vi "FindSimETH_CF.vi"(6 "COM":string, 8 "error in (no error)":errorcluster) -> (0 "error out":errorcluster, 1 "Pass":bool, 2 "CmdOut":string)   [LabVIEW 2013]
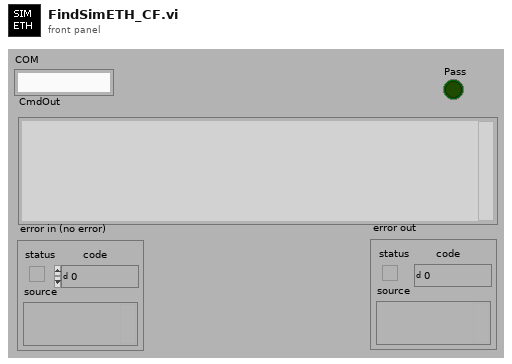
[diagram p1: front panel]
types:
  T1 = enum32{"invalid app kind", "Development System", "Run Time System", "Student Edition", "Embedded LabVIEW", "Evaluation", "Custom"}
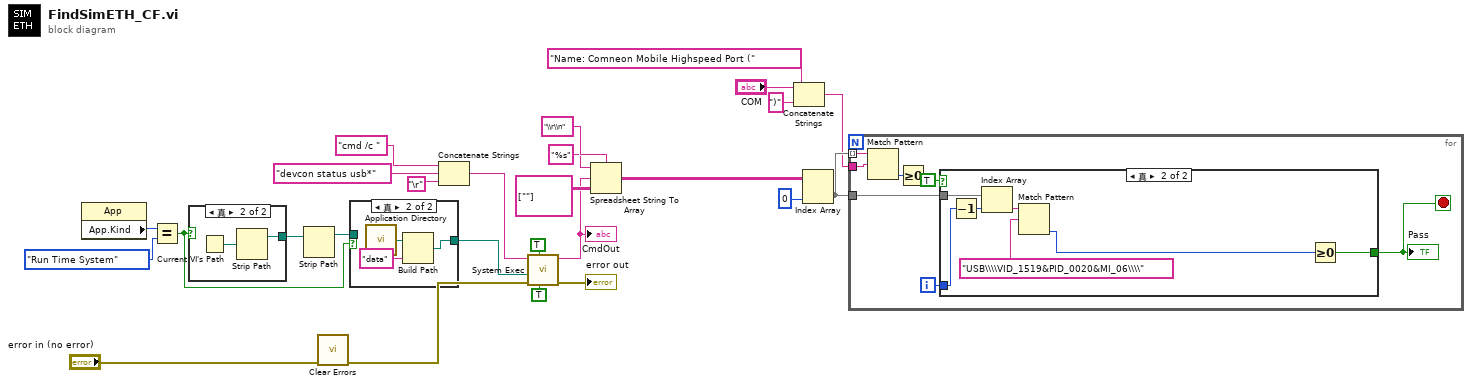
[diagram p0: block diagram]
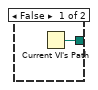
[diagram p3: hidden frame]
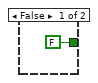
[diagram p4: hidden frame]
diagram:
  n1 = property class="App"() -> ("App.Kind"=w13:T1)  [unwired: 2 in, 2 out]
  n2 = Equal?(x=w13, y=T1."Run Time System") -> (x = y?=w4:bool)
  n3 = case shown="真" w4 {
    tunnel: [w27 w29] -> w12
    frame False {
      n4 = Current VI's Path() -> (path=w27:path)
    }
    frame True {
      n5 = Current VI's Path() -> (path=w28:path)
      n6 = Strip Path(path=w28) -> (stripped path=w29:path)  [unwired: 1 out]
    }
  }
  n7 = Strip Path(path=w12) -> (stripped path=w5:path)  [unwired: 1 out]
  n8 = call <vilib>:"Clear Errors.vi"("error in (no error)"="error in (no error)") -> ("error out"=w2:errorcluster)  [unwired: 6 in]
  n9 = case shown="真" w4 {
    tunnel: w5 -> [w30 _]
    tunnel: [w30 w31] -> w1
    frame False {
    }
    frame True {
      n10 = call <vilib>:"Application Directory.vi"() -> ("Application Directory"=w33:path)
      n11 = Build Path(base path=w33, name or relative path="data" ("名称或相对路径")) -> (appended path=w31:path)
    }
  }
  n12 = Concatenate Strings("cmd /c " ("command line"), "devcon status usb*" ("command"), "\r") -> (w24:string)
  n13 = call <vilib>:"System Exec.vi"("run minimized? (F)"=TRUE, "wait until completion? (T)"=TRUE, "error in (no error)"=w2, "working directory"=w1, "command line"=w24) -> ("error out"=→"error out":errorcluster, "standard output"=w15:string)  [unwired: 1 in, 4 out]
  "CmdOut" <- w15
  n14 = Spreadsheet String To Array(delimiter (Tab)="\\r\\n" ("格式字符串"), format string="%s" ("格式字符串"), spreadsheet string=w15, array type (2D Dbl)=string[][] [[""]]) -> (array=w17:string[][])
  n15 = Concatenate Strings("Name: Comneon Mobile Highspeed Port (" ("command line"), "COM", ")" ("字符串")) -> (w7:string)
  n16 = Index Array(array=w17, index (col)=0 ("索引 (行)")) -> (element=w10:string[])  [unwired: 1 in]
  n17 = for {
    tunnel: w10 -> [w40] mode=indexing
    tunnel: w7 -> [w39]
    tunnel: w10 -> [w37]
    i -> [w38]
    stop <- w35 stop-if-true
    n18 = Match Pattern(string=w40, regular expression=w39) -> (offset past match=w36:i32)  [unwired: 4 out]
    n19 = Greater Or Equal To 0?(x=w36) -> ()  [unwired: 1 out]
    n20 = case shown="真" TRUE {
      tunnel: w38 -> [_ w48]
      tunnel: w37 -> [_ w45]
      tunnel: [FALSE w44] -> w35
      frame False {
      }
      frame True {
        n21 = Decrement(x=w48) -> (x-1=w47:i32)
        n22 = Index Array(array=w45, index=w47) -> (element=w46:string)
        n23 = Match Pattern(string=w46, regular expression="USB\\\\VID_1519&PID_0020&MI_06\\\\" ("正则表达式")) -> (offset past match=w42:i32)  [unwired: 1 in, 3 out]
        n24 = Greater Or Equal To 0?(x=w42) -> (x >= 0?=w44:bool)
      }
    }
    "Pass" <- w35
  }
